vi "Configuration Convert 1.1 to 1.0.vi"(8 "error in (no error)":errorcluster, 11 "framework configuration 1.1":T2={"plugins"=[{"name"="Plugin", "components"=[], "cycle timing"={"priority"=10000, "decimation"=1, "offset"=0}, "threads"=[], "transfer groups"=[{"name"="Group", "direction"=0, "cycle timing"={"priority"=100, "decimation"=1, "offset"=0}, "thread index"=-1, "settings"=[], "transfers"=[{"name"="Transfer", "byte order"=0, "settings"=[], "channels"=[{"string offset"=0, "string data type"=2, "engine data type"=2, "name"="Channel", "settings"=[], "units"="V"}]}], "timeout behavior"=0}], "settings"=[]}]}) -> (0 "error out":errorcluster, 3 "framework configuration 1.0":T1)   [LabVIEW 2021, in "DSF Core.lvlib" / "Configuration Session.lvclass"]
uses:
  Configuration Session.lvclass
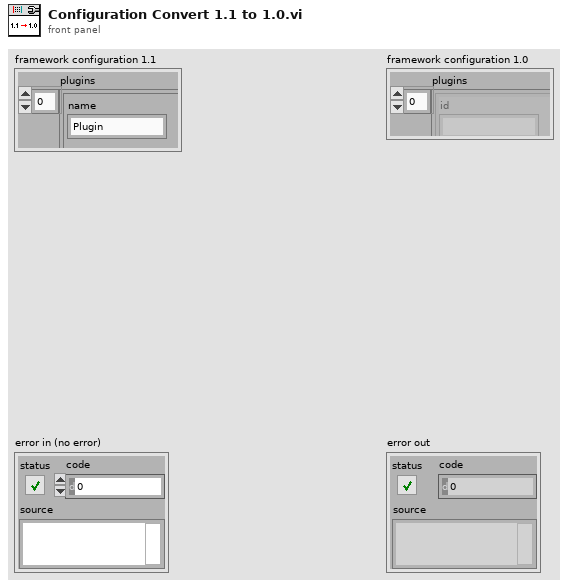
[diagram p1: front panel]
types:
  T1 = cluster{"plugins":cluster{"id":string, "values":cluster{"components":string[], "timing":cluster{"priority":u64, "decimation":u64, "offset":u64}, "group ids":string[], "settings id":string, "threads":cluster{"buffer converter settings":cluster{"key":string, "value":string}[], "transceiver settings":cluster{"key":string, "value":string}[], "custom settings":cluster{"key":string, "value":string}[], "processor":i32, "priority offset":i16}[]}}[], "groups":cluster{"id":string, "values":cluster{"direction":i32, "timing":cluster{"priority":u64, "decimation":u64, "offset":u64}, "transfer ids":string[], "settings id":string, "thread":i32, "timeout behavior":u8}}[], "transfers":cluster{"id":string, "values":cluster{"byte order":i32, "channel ids":string[], "settings id":string}}[], "channels":cluster{"id":string, "values":cluster{"string buffer offset":u64, "string data type":i32, "engine data type":i32, "settings id":string, "units":string}}[], "settings":cluster{"id":string, "values":cluster{"key":string, "value":string}[]}[]}
  T2 = cluster{"plugins":cluster{"name":string, "components":string[], "cycle timing":cluster{"priority":u64, "decimation":u64, "offset":u64}, "threads":cluster{"buffer converter settings":cluster{"key":string, "value":string}[], "transceiver settings":cluster{"key":string, "value":string}[], "custom settings":cluster{"key":string, "value":string}[], "processor":i32, "priority offset":i16}[], "transfer groups":cluster{"name":string, "direction":u8, "cycle timing":cluster{"priority":u64, "decimation":u64, "offset":u64}, "thread index":i32, "settings":cluster{"key":string, "value":string}[], "transfers":cluster{"name":string, "byte order":u8, "settings":cluster{"key":string, "value":string}[], "channels":cluster{"string offset":u64, "string data type":u8, "engine data type":u8, "name":string, "settings":cluster{"key":string, "value":string}[], "units":string}[]}[], "timeout behavior":u8}[], "settings":cluster{"key":string, "value":string}[]}[]}
  T3 = cluster{"components":string[], "timing":cluster{"priority":u64, "decimation":u64, "offset":u64}, "group ids":string[], "settings id":string, "threads":cluster{"buffer converter settings":cluster{"key":string, "value":string}[], "transceiver settings":cluster{"key":string, "value":string}[], "custom settings":cluster{"key":string, "value":string}[], "processor":i32, "priority offset":i16}[]}
  T4 = cluster{"id":string, "values":cluster{"components":string[], "timing":cluster{"priority":u64, "decimation":u64, "offset":u64}, "group ids":string[], "settings id":string, "threads":cluster{"buffer converter settings":cluster{"key":string, "value":string}[], "transceiver settings":cluster{"key":string, "value":string}[], "custom settings":cluster{"key":string, "value":string}[], "processor":i32, "priority offset":i16}[]}}
  T5 = cluster{"id":string, "values":cluster{"key":string, "value":string}[]}
  T6 = cluster{"direction":i32, "timing":cluster{"priority":u64, "decimation":u64, "offset":u64}, "transfer ids":string[], "settings id":string, "thread":i32, "timeout behavior":u8}
  T7 = cluster{"id":string, "values":cluster{"direction":i32, "timing":cluster{"priority":u64, "decimation":u64, "offset":u64}, "transfer ids":string[], "settings id":string, "thread":i32, "timeout behavior":u8}}
  T8 = cluster{"byte order":i32, "channel ids":string[], "settings id":string}
  T9 = cluster{"id":string, "values":cluster{"byte order":i32, "channel ids":string[], "settings id":string}}
  T10 = cluster{"string buffer offset":u64, "string data type":i32, "engine data type":i32, "settings id":string, "units":string}
  T11 = cluster{"id":string, "values":cluster{"string buffer offset":u64, "string data type":i32, "engine data type":i32, "settings id":string, "units":string}}
  T12 = cluster{"name":string, "components":string[], "cycle timing":cluster{"priority":u64, "decimation":u64, "offset":u64}, "threads":cluster{"buffer converter settings":cluster{"key":string, "value":string}[], "transceiver settings":cluster{"key":string, "value":string}[], "custom settings":cluster{"key":string, "value":string}[], "processor":i32, "priority offset":i16}[], "transfer groups":cluster{"name":string, "direction":u8, "cycle timing":cluster{"priority":u64, "decimation":u64, "offset":u64}, "thread index":i32, "settings":cluster{"key":string, "value":string}[], "transfers":cluster{"name":string, "byte order":u8, "settings":cluster{"key":string, "value":string}[], "channels":cluster{"string offset":u64, "string data type":u8, "engine data type":u8, "name":string, "settings":cluster{"key":string, "value":string}[], "units":string}[]}[], "timeout behavior":u8}[], "settings":cluster{"key":string, "value":string}[]}[]
  T13 = cluster{"priority":u64, "decimation":u64, "offset":u64}
  T14 = cluster{"buffer converter settings":cluster{"key":string, "value":string}[], "transceiver settings":cluster{"key":string, "value":string}[], "custom settings":cluster{"key":string, "value":string}[], "processor":i32, "priority offset":i16}[]
  T15 = cluster{"name":string, "direction":u8, "cycle timing":cluster{"priority":u64, "decimation":u64, "offset":u64}, "thread index":i32, "settings":cluster{"key":string, "value":string}[], "transfers":cluster{"name":string, "byte order":u8, "settings":cluster{"key":string, "value":string}[], "channels":cluster{"string offset":u64, "string data type":u8, "engine data type":u8, "name":string, "settings":cluster{"key":string, "value":string}[], "units":string}[]}[], "timeout behavior":u8}[]
  T16 = cluster{"name":string, "byte order":u8, "settings":cluster{"key":string, "value":string}[], "channels":cluster{"string offset":u64, "string data type":u8, "engine data type":u8, "name":string, "settings":cluster{"key":string, "value":string}[], "units":string}[]}[]
  T17 = cluster{"string offset":u64, "string data type":u8, "engine data type":u8, "name":string, "settings":cluster{"key":string, "value":string}[], "units":string}[]
  T18 = cluster{"id":string, "values":cluster{"key":string, "value":string}[]}[]
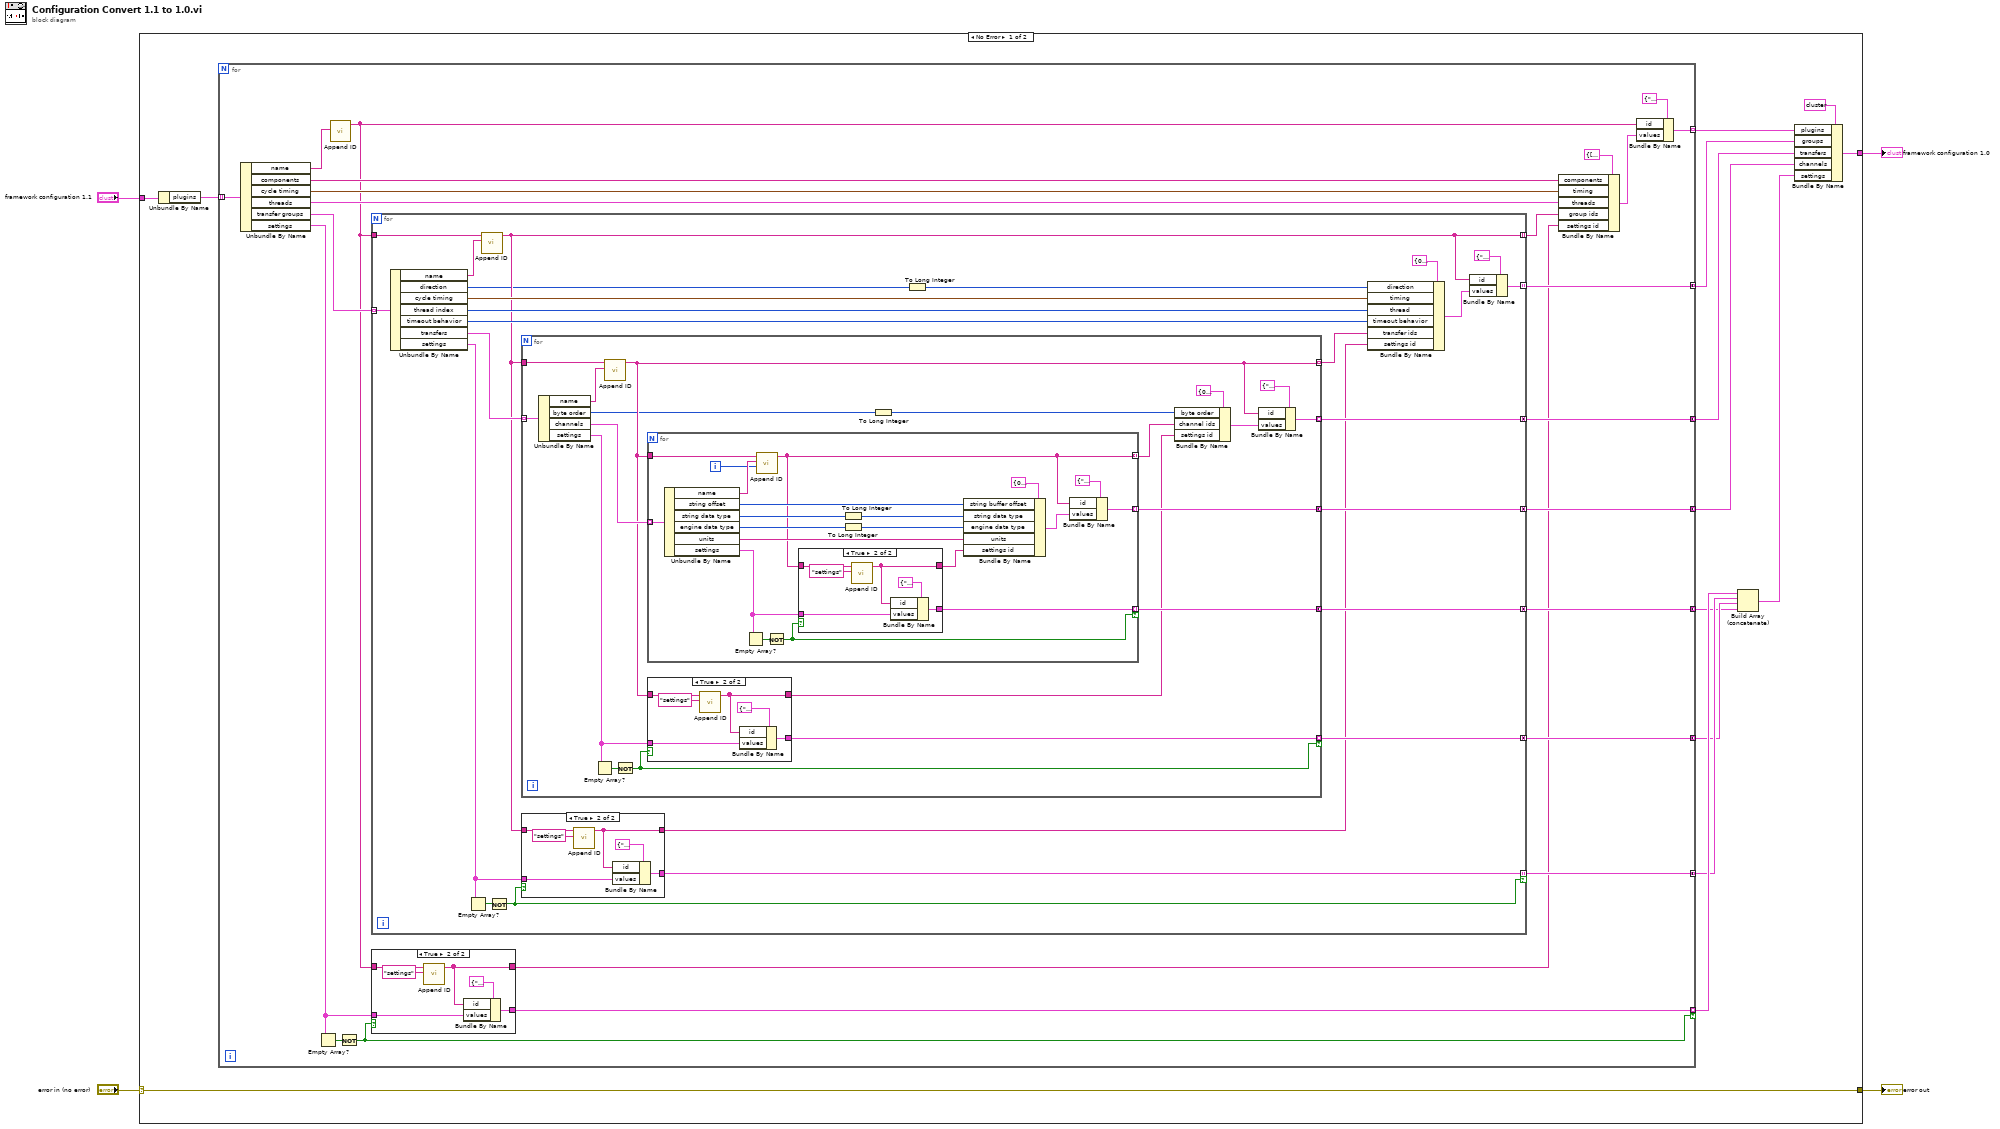
[diagram p0: block diagram]
diagram:
  n1 = case shown="No Error" "error in (no error)" {
    selector: "error in (no error)" -> [w17 w129]
    tunnel: [w17 w129] -> w4
    tunnel: [w18 _] -> w1
    tunnel: "framework configuration 1.1" -> [w16 _]
    frame No Error {
      n2 = Unbundle By Name(w16) -> ("plugins"=w15:T12)
      n3 = for {
        tunnel: w15 -> [w41] mode=indexing
        tunnel: [w40] -> w14 mode=indexing
        tunnel: [w33] -> w13 mode=concatenating
        tunnel: [w31] -> w12 mode=concatenating
        tunnel: [w30] -> w11 mode=concatenating
        tunnel: [w29] -> w7 mode=concatenating
        tunnel: [w25] -> w8 mode=concatenating
        tunnel: [w24] -> w9 mode=concatenating
        tunnel: [w23] -> w10 mode=indexing if=w22
        n4 = Unbundle By Name(w41) -> ("name"=w35:string, "components"=w38:string[], "cycle timing"=w37:T13, "threads"=w36:T14, "transfer groups"=w34:T15, "settings"=w27:cluster{"key":string, "value":string}[])
        n5 = Empty Array?(array=w27) -> (empty?=w28:bool)
        n6 = call "Append ID.vi"("name"=w35) -> ("appended id string"=w26:string)  [unwired: 10 in]
        n7 = Not(x=w28) -> (.not. x?=w22:bool)
        n8 = for {
          tunnel: w34 -> [w71] mode=indexing
          tunnel: w26 -> [w70]
          tunnel: [w68] -> w33 mode=indexing
          tunnel: [w56] -> w32 mode=indexing
          tunnel: [w61] -> w31 mode=concatenating
          tunnel: [w60] -> w30 mode=concatenating
          tunnel: [w59] -> w29 mode=concatenating
          tunnel: [w55] -> w25 mode=concatenating
          tunnel: [w54] -> w24 mode=indexing if=w53
          n9 = Unbundle By Name(w71) -> ("name"=w69:string, "direction"=w49:u8, "cycle timing"=w66:T13, "thread index"=w65:i32, "timeout behavior"=w64:u8, "transfers"=w63:T16, "settings"=w57:cluster{"key":string, "value":string}[])
          n10 = Empty Array?(array=w57) -> (empty?=w58:bool)
          n11 = call "Append ID.vi"("name"=w69, "initial id string (\"\")"=w70) -> ("appended id string"=w56:string)  [unwired: 9 in]
          n12 = Not(x=w58) -> (.not. x?=w53:bool)
          n13 = for {
            tunnel: w63 -> [w96] mode=indexing
            tunnel: w56 -> [w95]
            tunnel: [w86] -> w62 mode=indexing
            tunnel: [w92] -> w61 mode=indexing
            tunnel: [w89] -> w60 mode=concatenating
            tunnel: [w85] -> w55 mode=indexing if=w84
            tunnel: [w83] -> w59 mode=concatenating
            n14 = Unbundle By Name(w96) -> ("name"=w94:string, "byte order"=w79:u8, "channels"=w91:T17, "settings"=w87:cluster{"key":string, "value":string}[])
            n15 = Empty Array?(array=w87) -> (empty?=w88:bool)
            n16 = call "Append ID.vi"("name"=w94, "initial id string (\"\")"=w95) -> ("appended id string"=w86:string)  [unwired: 9 in]
            n17 = Not(x=w88) -> (.not. x?=w84:bool)
            n18 = for {
              tunnel: w86 -> [w122]
              tunnel: w91 -> [w121] mode=indexing
              tunnel: [w108] -> w90 mode=indexing
              tunnel: [w117] -> w89 mode=indexing
              tunnel: [w113] -> w83 mode=indexing if=w109
              i -> [w107]
              n19 = Unbundle By Name(w121) -> ("name"=w120:string, "string offset"=w118:u64, "string data type"=w116:u8, "engine data type"=w115:u8, "units"=w114:string, "settings"=w110:cluster{"key":string, "value":string}[])
              n20 = Empty Array?(array=w110) -> (empty?=w111:bool)
              n21 = call "Append ID.vi"("appended number (-1: none)"=w107, "name"=w120, "initial id string (\"\")"=w122) -> ("appended id string"=w108:string)  [unwired: 8 in]
              n22 = Not(x=w111) -> (.not. x?=w109:bool)
              n23 = case shown="True" w109 {
                tunnel: [_ w128] -> w113
                tunnel: w110 -> [_ w127]
                tunnel: w108 -> [_ w125]
                tunnel: [_ w124] -> w112
                frame False {
                }
                frame True {
                  n24 = call "Append ID.vi"("name"="settings", "initial id string (\"\")"=w125) -> ("appended id string"=w124:string)  [unwired: 9 in]
                  n25 = Bundle By Name(cluster=T5 {"id"="Settings", "values"=[{"key"="a", "value"="a"}]} ("settings"), "id"=w124, "values"=w127) -> (w128:T5)
                }
              }
              n26 = To Long Integer(number=w116) -> (32bit integer=w104:i32)
              n27 = To Long Integer(number=w115) -> (32bit integer=w103:i32)
              n28 = Bundle By Name(cluster=T10 {"string buffer offset"=0, "string data type"=0, "engine data type"=0, "settings id"="", "units"="V"} ("values"), "string buffer offset"=w118, "string data type"=w104, "engine data type"=w103, "units"=w114, "settings id"=w112) -> (w119:T10)
              n29 = Bundle By Name(cluster=T11 {"id"="Channel", "values"={"string buffer offset"=0, "string data type"=0, "engine data type"=0, "settings id"="", "units"="V"}} ("channel"), "id"=w108, "values"=w119) -> (w117:T11)
            }
            n30 = case shown="True" w84 {
              tunnel: [_ w102] -> w85
              tunnel: w87 -> [_ w101]
              tunnel: w86 -> [_ w99]
              tunnel: [_ w98] -> w82
              frame False {
              }
              frame True {
                n31 = call "Append ID.vi"("name"="settings", "initial id string (\"\")"=w99) -> ("appended id string"=w98:string)  [unwired: 9 in]
                n32 = Bundle By Name(cluster=T5 {"id"="Settings", "values"=[{"key"="a", "value"="a"}]} ("settings"), "id"=w98, "values"=w101) -> (w102:T5)
              }
            }
            n33 = To Long Integer(number=w79) -> (32bit integer=w78:i32)
            n34 = Bundle By Name(cluster=T8 {"byte order"=0, "channel ids"=["Channel"], "settings id"=""} ("values"), "byte order"=w78, "channel ids"=w90, "settings id"=w82) -> (w93:T8)
            n35 = Bundle By Name(cluster=T9 {"id"="Transfer", "values"={"byte order"=0, "channel ids"=["Channel"], "settings id"=""}} ("transfer"), "id"=w86, "values"=w93) -> (w92:T9)
          }
          n36 = case shown="True" w53 {
            tunnel: [_ w77] -> w54
            tunnel: w57 -> [_ w76]
            tunnel: w56 -> [_ w74]
            tunnel: [_ w73] -> w52
            frame False {
            }
            frame True {
              n37 = call "Append ID.vi"("name"="settings", "initial id string (\"\")"=w74) -> ("appended id string"=w73:string)  [unwired: 9 in]
              n38 = Bundle By Name(cluster=T5 {"id"="Settings", "values"=[{"key"="a", "value"="a"}]} ("settings"), "id"=w73, "values"=w76) -> (w77:T5)
            }
          }
          n39 = To Long Integer(number=w49) -> (32bit integer=w48:i32)
          n40 = Bundle By Name(cluster=T6 {"direction"=0, "timing"={"priority"=0, "decimation"=1, "offset"=0}, "transfer ids"=["Transfer"], "settings id"="", "thread"=0, "timeout behavior"=0} ("values"), "direction"=w48, "timing"=w66, "thread"=w65, "timeout behavior"=w64, "transfer ids"=w62, "settings id"=w52) -> (w67:T6)
          n41 = Bundle By Name(cluster=T7 {"id"="Group", "values"={"direction"=0, "timing"={"priority"=0, "decimation"=1, "offset"=0}, "transfer ids"=["Transfer"], "settings id"="", "thread"=0, "timeout behavior"=0}} ("group"), "id"=w56, "values"=w67) -> (w68:T7)
        }
        n42 = case shown="True" w22 {
          tunnel: [_ w47] -> w23
          tunnel: w27 -> [_ w46]
          tunnel: w26 -> [_ w44]
          tunnel: [_ w43] -> w21
          frame False {
          }
          frame True {
            n43 = call "Append ID.vi"("name"="settings", "initial id string (\"\")"=w44) -> ("appended id string"=w43:string)  [unwired: 9 in]
            n44 = Bundle By Name(cluster=T5 {"id"="Settings", "values"=[{"key"="a", "value"="a"}]} ("settings"), "id"=w43, "values"=w46) -> (w47:T5)
          }
        }
        n45 = Bundle By Name(cluster=T3 {"components"=[], "timing"={"priority"=1000, "decimation"=1, "offset"=0}, "group ids"=["Group"], "settings id"="", "threads"=[{"buffer converter settings"=[], "transceiver settings"=[], "custom settings"=[], "processor"=-2, "priority offset"=0}, {"buffer converter settings"=[], "transceiver settings"=[], "custom settings"=[], "processor"=-2, "priority offset"=0}]} ("values"), "components"=w38, "timing"=w37, "threads"=w36, "group ids"=w32, "settings id"=w21) -> (w39:T3)
        n46 = Bundle By Name(cluster=T4 {"id"="", "values"={"components"=[], "timing"={"priority"=0, "decimation"=0, "offset"=0}, "group ids"=[], "settings id"="", "threads"=[]}} ("plugins"), "id"=w26, "values"=w39) -> (w40:T4)
      }
      n47 = Build Array (concatenate)(w10, w9, w8, w7) -> (w6:T18)
      n48 = Bundle By Name(cluster=T1 {"plugins"=[{"id"="Test Plugin", "values"={"components"=[], "timing"={"priority"=1000, "decimation"=1, "offset"=0}, "group ids"=["Group"], "settings id"="", "threads"=[{"buffer converter settings"=[], "transceiver settings"=[], "custom settings"=[], "processor"=-2, "priority offset"=0}, {"buffer converter settings"=[], "transceiver settings"=[], "custom settings"=[], "processor"=-2, "priority offset"=0}]}}], "groups"=[{"id"="Group", "values"={"direction"=0, "timing"={"priority"=0, "decimation"=1, "offset"=0}, "transfer ids"=["Transfer"], "settings id"="", "thread"=0, "timeout behavior"=0}}], "transfers"=[{"id"="Transfer", "values"={"byte order"=0, "channel ids"=["Channel"], "settings id"=""}}], "channels"=[{"id"="Channel", "values"={"string buffer offset"=0, "string data type"=0, "engine data type"=0, "settings id"="", "units"="V"}}], "settings"=[{"id"="Settings", "values"=[{"key"="a", "value"="a"}]}]} ("framework configuration 1.0"), "plugins"=w14, "groups"=w13, "transfers"=w12, "channels"=w11, "settings"=w6) -> (w18:T1)
    }
    frame Error {
    }
  }
  "error out" <- w4
  "framework configuration 1.0" <- w1
